vi "ustawieniaRuchu.vi"(6 "error in":errorcluster, 7 "Lista komór":T1[](array[typedef]), 8 "Rodzaj akcji":T8=enum."Reset ramienia", 9 "LINX Resource in":T2) -> (0 "error out":errorcluster, 2 "Nowa lista komór":T1[](array[typedef]), 3 "LINX Resource out":T2)   [LabVIEW 2014]
uses:
  AkcjaRuchu.ctl
  <vilib>/MakerHub/LINX/Private/Type Defs/LINX Ref.ctl
  <vilib>/MakerHub/LINX/Private/Type Defs/Platform.ctl
  <vilib>/MakerHub/LINX/Private/Type Defs/Interface.ctl
  <vilib>/MakerHub/LINX/Private/Device/Type Defs/LINX Device Config.ctl
  <vilib>/MakerHub/LINX/Private/Device/Type Defs/TCP Config.ctl
  <vilib>/MakerHub/LINX/Private/Device/Type Defs/Channels.ctl
  wykonajRuchVIs/parametryKomorVIs/WyborKomory.ctl
  AkcjaGFV.ctl
  <vilib>/MakerHub/LINX/Public/Utilities/Open Local.vi
  <vilib>/MakerHub/LINX/LMH-LINX.lvlib
  <vilib>/MakerHub/LINX/Private/Device/Device.lvlib
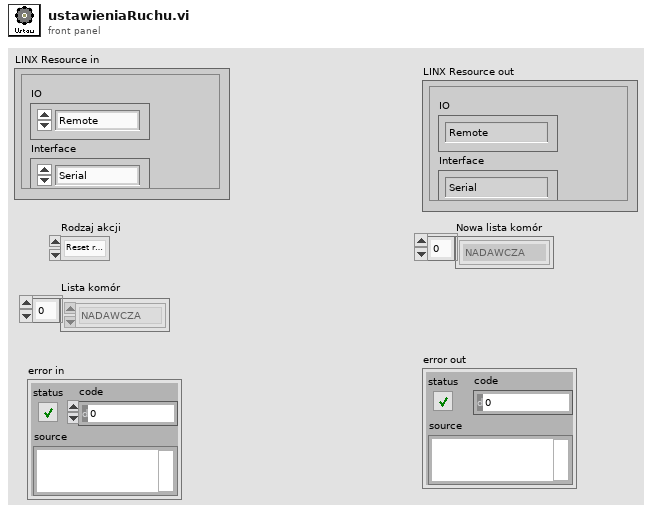
[diagram p1: front panel]
types:
  T1 = typedef "WyborKomory.ctl" = enum16{"NADAWCZA", "ODBIORCZA"}
  T2 = typedef "LMH-LINX.lvlib/LINX Ref.ctl" = cluster{"IO":T3, "Interface":T4, "LINX Device Config":T5}
  T3 = typedef "LMH-LINX.lvlib/Platform.ctl" = enum16{"Remote", "Local"}
  T4 = typedef "LMH-LINX.lvlib/Interface.ctl" = enum16{"Serial", "TCP"}
  T5 = typedef "LMH-LINX.lvlib/Device.lvlib/LINX Device Config.ctl" = cluster{"Interface":T4, "COM Port":refnum<visa-resource-name>, "TCP Configuration":T6, "Device Family":u8, "Device ID":u8, "Device Name":string, "TCP Ref":refnum<k5>, "Channels":T7}
  T6 = typedef "LMH-LINX.lvlib/Device.lvlib/TCP Config.ctl" = cluster{"IP Address":string, "Port":u16}
  T7 = typedef "LMH-LINX.lvlib/Channels.ctl" = cluster{"DI":u8[], "DO":u8[], "AI":u8[], "AO":u8[], "PWM":u8[], "QE":u8[], "UART":u8[], "I2C 2":u8[], "SPI":u8[], "CAN":u8[], "Servo":u8[], "AI Ref (V)":dbl, "AI Resolution (Bits)":u8, "AO Ref (V)":dbl, "AO Resolution (Bits)":u8}
  T8 = typedef "AkcjaRuchu.ctl" = enum16{"Init", "Reset ramienia", "Przygotuj listê", "SprawdŸ", "Koniec"}
  T9 = typedef "AkcjaGFV.ctl" = enum16{"Czytaj", "Zapisz", "Reset"}
  T10 = typedef "WyjsciaParametry.ctl" = cluster{"Nad. lewo":bool, "Nad.  prawo":bool, "Nad.  gora":bool, "Nad. do³":bool, "Dzialanie":bool, "Pomiar":bool, "Odb. lewo":bool, "Odb.  prawo":bool, "Odb.  gora":bool, "Odb. dol":bool, "Pozostalo punktow":i32, "Nad. elewacja":i32, "Nad. azymut":i32, "Odb. elewacja":i32, "Odb. azymut":i32, "TCP Error":bool, "TCP Error Code":i32, "LINX Error":bool, "LINX Error Code":i32, "Nastepny elewacja":i32, "Nastepny azymut":i32, "Coords Error":bool, "Inicjalizacja pozycji":bool, "Generator Error":bool, "Error Code":i32}
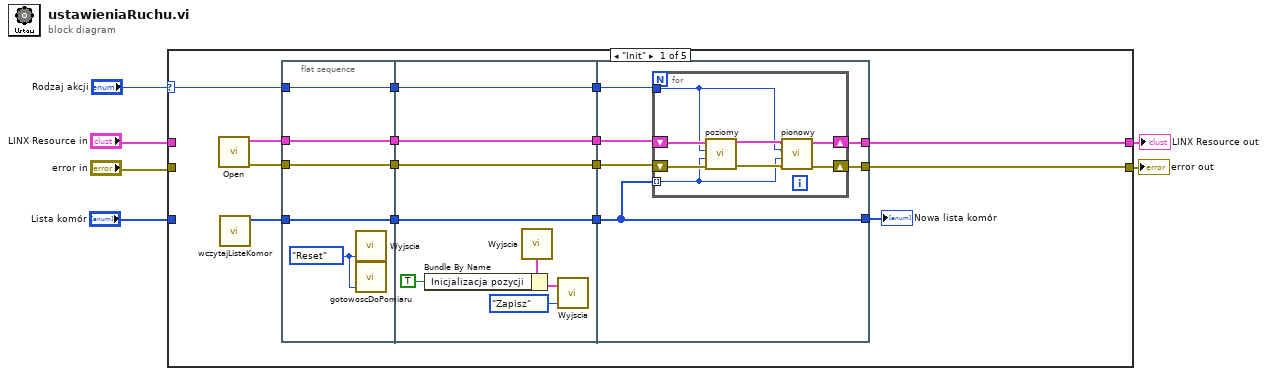
[diagram p0: block diagram]
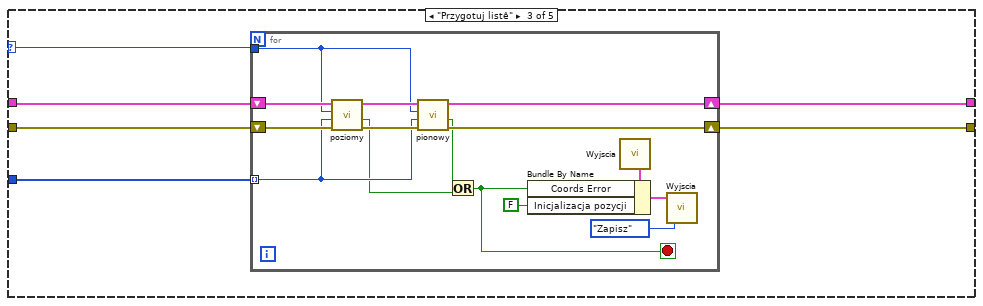
[diagram p3: hidden frame]
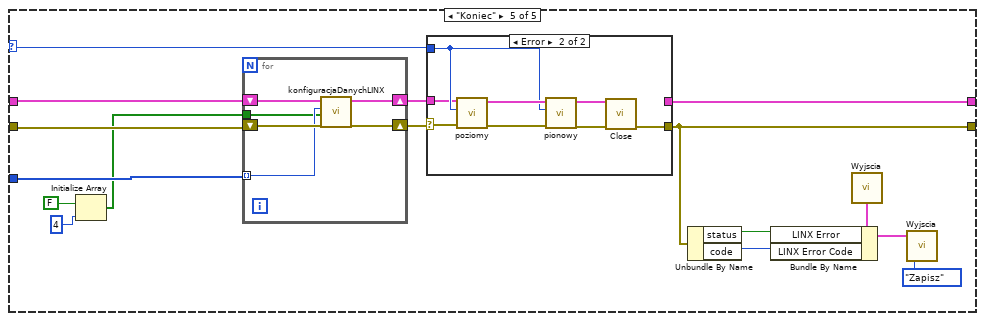
[diagram p5: hidden frame]
diagram:
  n1 = case shown="\"Init\"" "Rodzaj akcji" {
    selector: "Rodzaj akcji" -> [w20 _ w53 _ w88]
    tunnel: "LINX Resource in" -> [_ w50 w54 w73 w86]
    tunnel: "error in" -> [_ w49 w55 w72 w85]
    tunnel: [w21 w50 w56 w73 w89] -> w4
    tunnel: [w9 w49 w51 w72 w74] -> w1
    tunnel: "Lista komór" -> [_ _ w52 _ w84]
    frame "Init" {
      n2 = call-poly <vilib>:"Open.vi"() -> ("Error Out"=w18:errorcluster, "LINX Resource"=w19:T2)  [unwired: 9 in, 1 out]
      n3 = call "wczytajListeKomor.vi"() -> ("Lista komór"=w8:T1[])  [unwired: 11 in]
      n4 = flat-sequence {
        tunnel: w18 -> [w23]
        tunnel: w19 -> [w24]
        tunnel: w8 -> [w25]
        tunnel: w20 -> [w26]
        tunnel: [w26] -> w17
        tunnel: [w25] -> w15
        tunnel: [w24] -> w13
        tunnel: [w23] -> w11
        tunnel: w17 -> [w34]
        tunnel: [w34] -> w16
        tunnel: w15 -> [w33]
        tunnel: [w33] -> w14
        tunnel: w13 -> [w32]
        tunnel: [w32] -> w12
        tunnel: w11 -> [w31]
        tunnel: [w31] -> w10
        tunnel: [w40] -> w21
        tunnel: [w38] -> w9
        tunnel: w16 -> [w39]
        tunnel: w14 -> [w35]
        tunnel: w12 -> [w37]
        tunnel: w10 -> [w36]
        tunnel: [w35] -> w7
        frame #0 {
          w22 = AkcjaGFV."Reset" ("Akcja")
          n5 = call "Wyjscia.vi"("Akcja"=w22) -> ()  [unwired: 4 in, 1 out]
          n6 = call "gotowoscDoPomiaru.vi"("Akcja"=w22) -> ()  [unwired: 4 in, 1 out]
        }
        frame #1 {
          n7 = call "Wyjscia.vi"() -> ("Wyjœcie"=w30:T10)  [unwired: 5 in]
          n8 = Bundle By Name(cluster=w30, "Inicjalizacja pozycji"=TRUE) -> (w28:T10)
          n9 = call "Wyjscia.vi"("Akcja"=AkcjaGFV."Zapisz", "Wejœcie"=w28) -> ()  [unwired: 3 in, 1 out]
        }
        frame #2 {
          n10 = for {
            tunnel: w39 -> [w42]
            shift-right: [w44] -> w40
            shift-left: w37 -> [w46]
            shift-right: [w43] -> w38
            shift-left: w36 -> [w45]
            tunnel: w35 -> [w41] mode=indexing
            n11 = call "poziomy.vi"("error in (no error)"=w45, "Wybór komory"=w41, "Akcja"=w42, "LINX Resource in"=w46) -> ("error out"=w47:errorcluster, "LINX Resource out"=w48:T2)  [unwired: 2 in, 2 out]
            n12 = call "pionowy.vi"("error in"=w47, "Wybór komory"=w41, "Akcja"=w42, "LINX Resource in"=w48) -> ("error out"=w43:errorcluster, "LINX Resource out"=w44:T2)  [unwired: 2 in, 2 out]
          }
        }
      }
      "Nowa lista komór" <- w7
    }
    frame "Reset ramienia" {
    }
    frame "Przygotuj listê" {
      n13 = for {
        tunnel: w53 -> [w65]
        shift-right: [w68] -> w51
        shift-left: w55 -> [w67]
        shift-right: [w69] -> w56
        shift-left: w54 -> [w66]
        tunnel: w52 -> [w64] mode=indexing
        stop <- w58 stop-if-true
        n14 = call "poziomy.vi"("error in (no error)"=w67, "Wybór komory"=w64, "Akcja"=w65, "LINX Resource in"=w66) -> ("error out"=w70:errorcluster, "KONIEC"=w62:bool, "LINX Resource out"=w71:T2)  [unwired: 2 in, 1 out]
        n15 = call "pionowy.vi"("error in"=w70, "Wybór komory"=w64, "Akcja"=w65, "LINX Resource in"=w71) -> ("error out"=w68:errorcluster, "KONIEC"=w63:bool, "LINX Resource out"=w69:T2)  [unwired: 2 in, 1 out]
        n16 = Or(x=w63, y=w62) -> (x .or. y?=w58:bool)
        n17 = call "Wyjscia.vi"() -> ("Wyjœcie"=w60:T10)  [unwired: 5 in]
        n18 = Bundle By Name(cluster=w60, "Coords Error"=w58, "Inicjalizacja pozycji"=FALSE) -> (w61:T10)
        n19 = call "Wyjscia.vi"("Akcja"=AkcjaGFV."Zapisz", "Wejœcie"=w61) -> ()  [unwired: 3 in, 1 out]
      }
    }
    frame "SprawdŸ" {
    }
    frame "Koniec" {
      n20 = Initialize Array(FALSE, 4 ("dimension size")) -> (w81:bool[])
      n21 = for {
        shift-right: [w105] -> w87
        shift-left: w86 -> [w103]
        shift-right: [w104] -> w75
        shift-left: w85 -> [w102]
        tunnel: w84 -> [w101] mode=indexing
        tunnel: w81 -> [w100]
        n22 = call "konfiguracjaDanychLINX.vi"("Error In"=w102, "Kierunki"=w100, "Wybór komory"=w101, "LINX Resource"=w103) -> ("Error Out"=w104:errorcluster, "LINX Out"=w105:T2)  [unwired: 6 in]
      }
      n23 = case shown="Error" w75 {
        selector: w75 -> [w90 w95]
        tunnel: [w91 _] -> w89
        tunnel: [w90 w93] -> w74
        tunnel: w88 -> [_ w97]
        tunnel: w87 -> [w91 w96]
        frame No Error {
        }
        frame Error {
          n24 = call "poziomy.vi"("error in (no error)"=w95, "Akcja"=w97, "LINX Resource in"=w96) -> ("error out"=w98:errorcluster, "LINX Resource out"=w99:T2)  [unwired: 3 in, 2 out]
          n25 = call "pionowy.vi"("error in"=w98, "Akcja"=w97, "LINX Resource in"=w99) -> ("error out"=w92:errorcluster, "LINX Resource out"=w94:T2)  [unwired: 3 in, 2 out]
          n26 = call <vilib>:"Close.vi"("Error In"=w92, "LINX Resource"=w94) -> ("Error Out"=w93:errorcluster)  [unwired: 9 in]
        }
      }
      n27 = Unbundle By Name(w74) -> ("status"=w79:bool, "code"=w80:i32)
      n28 = call "Wyjscia.vi"() -> ("Wyjœcie"=w77:T10)  [unwired: 5 in]
      n29 = Bundle By Name(cluster=w77, "LINX Error"=w79, "LINX Error Code"=w80) -> (w76:T10)
      n30 = call "Wyjscia.vi"("Akcja"=AkcjaGFV."Zapisz", "Wejœcie"=w76) -> ()  [unwired: 3 in, 1 out]
    }
  }
  "error out" <- w1
  "LINX Resource out" <- w4
